vi "crc32.vi"(4 "Reflect Output? (T)":bool=TRUE, 6 "Reflect Input? (T)":bool=TRUE, 8 "Xor Out (0xFFFFFFFF)":u32=4294967295 format="%08x", 9 "Poly (0x04C11DB7)":u32=79764919 format="%08x", 10 "Init (0xFFFFFFFF)":u32=4294967295 format="%08x", 11 "Data in":string) -> (3 "CRC-32":u32 format="%08x")   [LabVIEW 2022 SP3, in "LabVIEW-Hashlib.lvlib"]
doc: "Calculates a 32-bit Cyclic Redundancy Check (CRC-32) for various algorithms."
uses:
  LabVIEW-Hashlib.lvlib
panel:
  # "Data = \"123456789\"\n\nAlgorithm     CRC-32     Poly       Init       RefIn RefOut XorOut\nCRC-32        0xCBF43926 0x04C11DB7 0xFFFFFFFF true  true   0xFFFFFFFF\nCRC-32/BZIP2  0xFC891918 0x04C11DB7 0xFFFFFFFF false false  0xFFFFFFFF\nCRC-32C       0xE3069283 0x1EDC6F41 0xFFFFFFFF true  true   0xFFFFFFFF\nCRC-32D       0x87315576 0xA833982B 0xFFFFFFFF true  true   0xFFFFFFFF\nCRC-32/JAMCRC 0x340BC6D9 0x04C11DB7 0xFFFFFFFF true  true   0x00000000\nCRC-32/MPEG-2 0x0376E6E7 0x04C11DB7 0xFFFFFFFF false false  0x00000000\nCRC-32/POSIX  0x765E7680 0x04C11DB7 0x00000000 false false  0xFFFFFFFF\nCRC-32Q       0x3010BF7F 0x814141AB 0x00000000 false false  0x00000000\nCRC-32/XFER   0xBD0BE338 0x000000AF 0x00000000 false false  0x00000000\n\nSource: https://crccalc.com/"
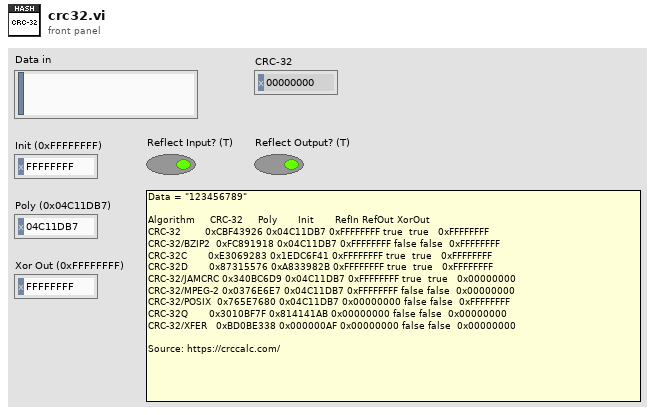
[diagram p1: front panel]
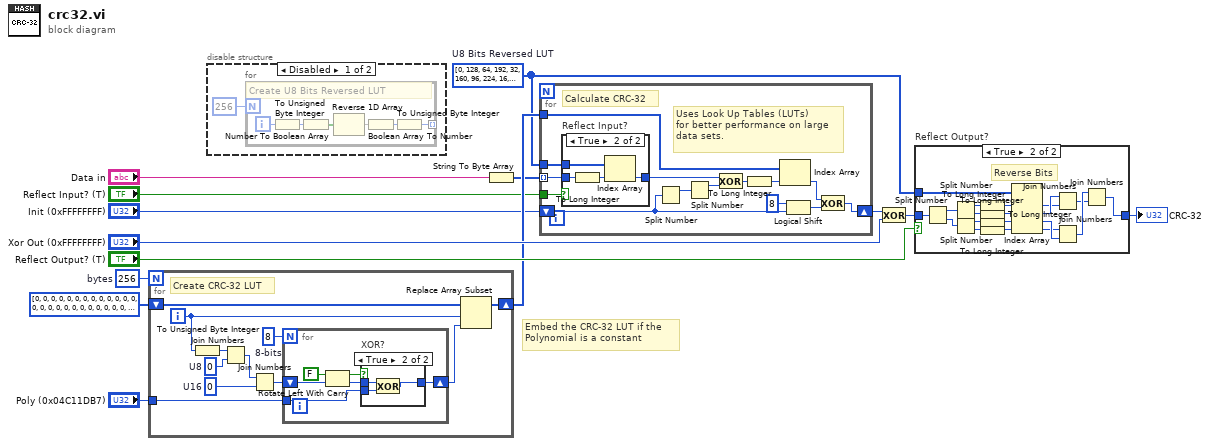
[diagram p0: block diagram]
diagram:
  w3 = u8[] [0, 128, 64, 192, 32, 160, 96, 224, 16, 144, 80, 208, 48, 176, 112, 240, 8, 136, 72, 200, 40, 168, 104, 232, 24, 152, 88, 216, 56, 184, 120, 248, 4, 132, 68, 196, 36, 164, 100, 228, 20, 148, 84, 212, 52, 180, 116, 244, 12, 140, 76, 204, 44, 172, 108, 236, 28, 156, 92, 220, 60, 188, 124, 252, 2, 130, 66, 194, 34, 162, 98, 226, 18, 146, 82, 210, 50, 178, 114, 242, 10, 138, 74, 202, 42, 170, 106, 234, 26, 154, 90, 218, 58, 186, 122, 250, 6, 134, 70, 198, 38, 166, 102, 230, 22, 150, 86, 214, 54, 182, 118, 246, 14, 142, 78, 206, 46, 174, 110, 238, 30, 158, 94, 222, 62, 190, 126, 254, 1, 129, 65, 193, 33, 161, 97, 225, 17, 145, 81, 209, 49, 177, 113, 241, 9, 137, 73, 201, 41, 169, 105, 233, 25, 153, 89, 217, 57, 185, 121, 249, 5, 133, 69, 197, 37, 165, 101, 229, 21, 149, 85, 213, 53, 181, 117, 245, 13, 141, 77, 205, 45, 173, 109, 237, 29, 157, 93, 221, 61, 189, 125, 253, 3, 131, 67, 195, 35, 163, 99, 227, 19, 147, 83, 211, 51, 179, 115, 243, 11, 139, 75, 203, 43, 171, 107, 235, 27, 155, 91, 219, 59, 187, 123, 251, 7, 135, 71, 199, 39, 167, 103, 231, 23, 151, 87, 215, 55, 183, 119, 247, 15, 143, 79, 207, 47, 175, 111, 239, 31, 159, 95, 223, 63, 191, 127, 255]  # U8 Bits Reversed LUT
  w4 = 256  # bytes
  # "Embed the CRC-32 LUT if the\nPolynomial is a constant"
  n1 = for {
    N: w4 -> [_]
    tunnel: "Poly (0x04C11DB7)" -> [w23]
    shift-right: [w19] -> w9
    shift-left: u32[] [0, 0, 0, 0, 0, 0, 0, 0, 0, 0, 0, 0, 0, 0, 0, 0, 0, 0, 0, 0, 0, 0, 0, 0, 0, 0, 0, 0, 0, 0, 0, 0, 0, 0, 0, 0, 0, 0, 0, 0, 0, 0, 0, 0, 0, 0, 0, 0, 0, 0, 0, 0, 0, 0, 0, 0, 0, 0, 0, 0, 0, 0, 0, 0, 0, 0, 0, 0, 0, 0, 0, 0, 0, 0, 0, 0, 0, 0, 0, 0, 0, 0, 0, 0, 0, 0, 0, 0, 0, 0, 0, 0, 0, 0, 0, 0, 0, 0, 0, 0, 0, 0, 0, 0, 0, 0, 0, 0, 0, 0, 0, 0, 0, 0, 0, 0, 0, 0, 0, 0, 0, 0, 0, 0, 0, 0, 0, 0, 0, 0, 0, 0, 0, 0, 0, 0, 0, 0, 0, 0, 0, 0, 0, 0, 0, 0, 0, 0, 0, 0, 0, 0, 0, 0, 0, 0, 0, 0, 0, 0, 0, 0, 0, 0, 0, 0, 0, 0, 0, 0, 0, 0, 0, 0, 0, 0, 0, 0, 0, 0, 0, 0, 0, 0, 0, 0, 0, 0, 0, 0, 0, 0, 0, 0, 0, 0, 0, 0, 0, 0, 0, 0, 0, 0, 0, 0, 0, 0, 0, 0, 0, 0, 0, 0, 0, 0, 0, 0, 0, 0, 0, 0, 0, 0, 0, 0, 0, 0, 0, 0, 0, 0, 0, 0, 0, 0, 0, 0, 0, 0, 0, 0, 0, 0, 0, 0, 0, 0, 0, 0, 0, 0, 0, 0, 0, 0] -> [w22]
    i -> [w21]
    w15 = u16 0  # U16
    w24 = 8  # 8-bits
    w25 = u8 0  # U8
    # "Create CRC-32 LUT"
    n2 = To Unsigned Byte Integer(number=w21) -> (unsigned 8bit integer=w18:u8)
    n3 = Join Numbers(hi=w18, lo=w25) -> ((hi.lo)=w17:u16)
    n4 = Join Numbers(hi=w17, lo=w15) -> ((hi.lo)=w16:u32)
    n5 = for {
      N: w24 -> [_]
      shift-right: [w27] -> w20
      shift-left: w16 -> [w31]
      tunnel: w23 -> [w28]
      n6 = Rotate Left With Carry(2:w31, 3:FALSE ("carry")) -> (0:w29:u32, 1:w26:bool)
      n7 = case "XOR?" shown="True" w26 {
        tunnel: w29 -> [w32 w35]
        tunnel: w28 -> [_ w34]
        tunnel: [w32 w33] -> w27
        frame False {
        }
        frame True {
          n8 = Exclusive Or(1:w34, 2:w35) -> (0:w33:u32)
        }
      }
    }
    n9 = Replace Array Subset(array=w22, new element=w20, index=w21) -> (w19:u32[])
  }
  n10 = disable-structure shown="Disabled" {
    frame Disabled {
      n11 = for {
        N: 256 -> [_]
        tunnel: [w37] -> _ mode=indexing
        i -> [w42]
        # "Create U8 Bits Reversed LUT"
        n12 = To Unsigned Byte Integer(number=w42) -> (unsigned 8bit integer=w41:u8)
        n13 = Number To Boolean Array(number=w41) -> (Boolean array=w40:bool[])
        n14 = Reverse 1D Array(array=w40) -> (reversed array=w39:bool[])
        n15 = Boolean Array To Number(Boolean array=w39) -> (number=w38:u32)
        n16 = To Unsigned Byte Integer(number=w38) -> (unsigned 8bit integer=w37:u8)
      }
    }
    frame Enabled {
    }
  }
  n17 = String To Byte Array(string="Data in") -> (unsigned byte array=w8:u8[])
  n18 = for {
    shift-right: [w48] -> w2
    shift-left: "Init (0xFFFFFFFF)" -> [w52]
    tunnel: w8 -> [w45] mode=indexing
    tunnel: w9 -> [w53]
    tunnel: "Reflect Input? (T)" -> [w44]
    tunnel: w3 -> [w47]
    # "Uses Look Up Tables (LUTs)\nfor better performance on large\ndata sets."
    # "Calculate CRC-32"
    n19 = case "Reflect Input?" shown="True" w44 {
      tunnel: w45 -> [w57 w61]
      tunnel: w47 -> [_ w59]
      tunnel: [w57 w58] -> w46
      frame False {
      }
      frame True {
        n20 = To Long Integer(number=w61) -> (32bit integer=w60:i32)
        n21 = Index Array(array=w59, index=w60) -> (element=w58:u8)
      }
    }
    n22 = Split Number(x=w52) -> (hi(x)=w56:u16)  [unwired: 1 out]
    n23 = Split Number(x=w56) -> (hi(x)=w43:u8)  [unwired: 1 out]
    n24 = Exclusive Or(1:w43, 2:w46) -> (0:w55:u8)
    n25 = To Long Integer(number=w55) -> (32bit integer=w54:i32)
    n26 = Index Array(array=w53, index=w54) -> (element=w49:u32)
    n27 = Logical Shift(y=i16 8, x=w52) -> (x << y=w50:u32)
    n28 = Exclusive Or(1:w50, 2:w49) -> (0:w48:u32)
  }
  n29 = Exclusive Or(1:"Xor Out (0xFFFFFFFF)", 2:w2) -> (0:w10:u32)
  n30 = case "Reflect Output?" shown="True" "Reflect Output? (T)" {
    tunnel: w10 -> [w62 w81]
    tunnel: [w62 w63] -> w14
    tunnel: w3 -> [_ w79]
    frame False {
    }
    frame True {
      # "Reverse Bits"
      n31 = Split Number(x=w81) -> (hi(x)=w80:u16, lo(x)=w76:u16)
      n32 = Split Number(x=w80) -> (hi(x)=w73:u8, lo(x)=w72:u8)
      n33 = Split Number(x=w76) -> (hi(x)=w71:u8, lo(x)=w70:u8)
      n34 = To Long Integer(number=w73) -> (32bit integer=w78:i32)
      n35 = To Long Integer(number=w72) -> (32bit integer=w77:i32)
      n36 = To Long Integer(number=w71) -> (32bit integer=w69:i32)
      n37 = To Long Integer(number=w70) -> (32bit integer=w68:i32)
      n38 = Index Array(array=w79, index #1=w78, index #2=w77, index #3=w69, index #4=w68) -> (element #1=w74:u8, element #2=w75:u8, element #3=w67:u8, element #4=w66:u8)
      n39 = Join Numbers(hi=w75, lo=w74) -> ((hi.lo)=w64:u16)
      n40 = Join Numbers(hi=w66, lo=w67) -> ((hi.lo)=w65:u16)
      n41 = Join Numbers(hi=w65, lo=w64) -> ((hi.lo)=w63:u32)
    }
  }
  "CRC-32" <- w14
